vi "Frisbee Joystick.vi"() -> (3 "Value":bool)   [LabVIEW 2012]
uses:
  Users/developer/Desktop/Post TCNJ/Robot Global Data.vi
panel:
  out "s? t:f":dbl
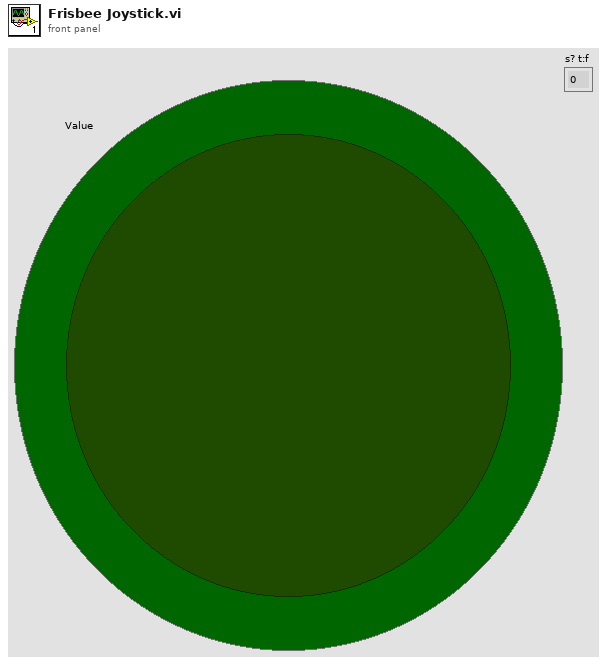
[diagram p1: front panel]
types:
  T1 = cluster{"Driver Station Digital Input (1-8)[0]":bool, "Driver Station Digital Input (1-8)[1]":bool, "Driver Station Digital Input (1-8)[2]":bool, "Driver Station Digital Input (1-8)[3]":bool, "Driver Station Digital Input (1-8)[4]":bool, "Driver Station Digital Input (1-8)[5]":bool, "Driver Station Digital Input (1-8)[6]":bool, "Driver Station Digital Input (1-8)[7]":bool, "Driver Station Digital Input (1-8)[8]":bool}
  T2 = typedef "WPI_DigitalInputDevRef.ctl" = cluster{"DevStatus":errorcluster, "DIO Channel":T3, "Digital Module":T4}
  T3 = typedef "FPGA_DIOChannel.ctl" = enum8{"DIO 1", "DIO 2", "DIO 3", "DIO 4", "DIO 5", "DIO 6", "DIO 7", "DIO 8", "DIO 9", "DIO 10", "DIO 11", "DIO 12", "DIO 13", "DIO 14", "Invalid"}
  T4 = typedef "FPGA_TypedefDigitalModule.ctl" = enum16{"Digital Module 1", "Digital Module 2"}
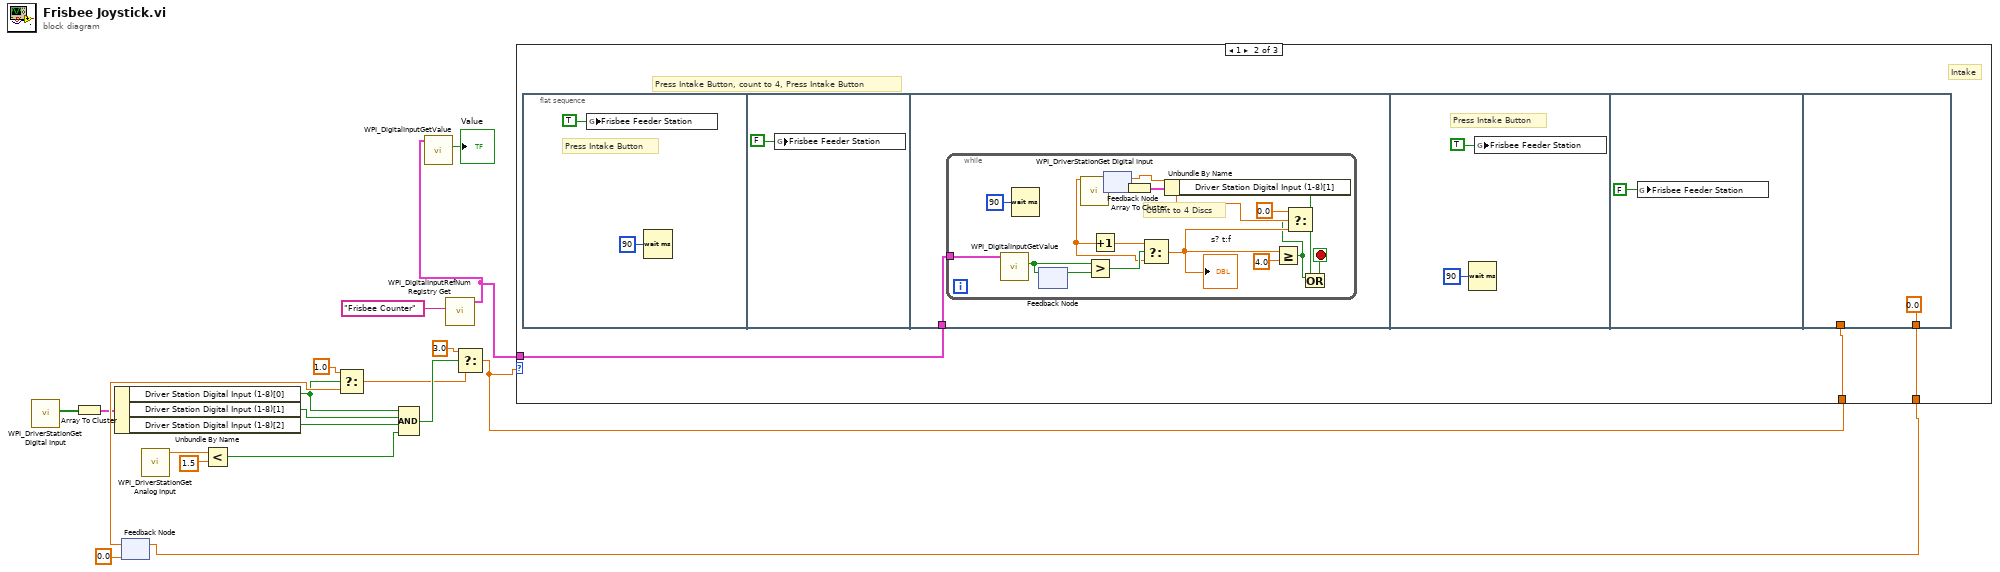
[diagram p0: block diagram]
diagram:
  n1 = call <vilib>:"WPI_DriverStationGet Digital Input.vi"() -> ("Driver Station Digital Input (1-8)"=w4:bool[])  [unwired: 11 in]
  n2 = Array To Cluster(array=w4) -> (cluster=w3:T1)
  n3 = Unbundle By Name(w3) -> ("Driver Station Digital Input (1-8)[0]"=w9:bool, "Driver Station Digital Input (1-8)[1]"=w17:bool, "Driver Station Digital Input (1-8)[2]"=w2:bool)
  n4 = feedback #1(0.0 ("t")) -> (w13:dbl)
  n5 = call <vilib>:"WPI_DriverStationGet Analog Input.vi"() -> ("Analog 1 (V)"=w5:dbl)  [unwired: 8 in, 3 out]
  n6 = Less?(x=w5, y=1.5) -> (x < y?=w7:bool)
  n7 = Select(t=1.0, s=w9, f=w13) -> (s? t:f=w1:dbl)
  n8 = Compound Arithmetic op=AND(w9, w17, w2, w7) -> (w8:bool)
  n9 = call <vilib>:"WPI_DigitalInputRefNum Registry Get.vi"("refnum name"="Frisbee Counter") -> ("DigitalInputDevRef"=w15:T2)  [unwired: 9 in, 1 out]
  n10 = call <vilib>:"WPI_DigitalInputGetValue.vi"("DigitalInputDevRef"=w15) -> ("Value"=→"Value":bool)  [unwired: 8 in, 2 out]
  n11 = Select(t=3.0, s=w8, f=w1) -> (s? t:f=w18:dbl)
  n12 = case shown="1" w18 {
    tunnel: w15 -> [_ w23 _]
    tunnel: w18 -> [w20 w22 w48]
    tunnel: [w20 w21 w48] -> w19
    frame 0, Default {
      # "Waiting For Signal."
      # "Do Nothing"
    }
    frame 1 {
      # "Press Intake Button, count to 4, Press Intake Button"
      # "Intake"
      n13 = flat-sequence {
        tunnel: w23 -> [w27]
        tunnel: w22 -> [_]
        tunnel: [0.0 ("t")] -> w21
        frame #0 {
          # "Press Intake Button"
          n14 = global write "Robot Global Data.vi" "Frisbee Feeder Station"(TRUE) -> ()
          n15 = Wait (ms)(milliseconds to wait=u32 90) -> ()  [unwired: 1 out]
        }
        frame #1 {
          n16 = global write "Robot Global Data.vi" "Frisbee Feeder Station"(FALSE) -> ()
        }
        frame #2 {
          n17 = while {
            tunnel: w27 -> [w39]
            stop <- w28 stop-if-true
            # "Count to 4 Discs"
            n18 = call <vilib>:"WPI_DigitalInputGetValue.vi"("DigitalInputDevRef"=w39) -> ("Value"=w40:bool)  [unwired: 8 in, 2 out]
            n19 = Wait (ms)(milliseconds to wait=u32 90) -> ()  [unwired: 1 out]
            n20 = feedback #2() -> (w41:bool)  [unwired: 1 in]
            n21 = feedback-in #2(w40) -> ()
            n22 = call <vilib>:"WPI_DriverStationGet Digital Input.vi"() -> ("Driver Station Digital Input (1-8)"=w32:bool[])  [unwired: 11 in]
            n23 = Greater?(x=w40, y=w41) -> (0:w43:bool)
            n24 = feedback #3() -> (w36:dbl)  [unwired: 1 in]
            n25 = Increment(x=w36) -> (x+1=w42:dbl)
            n26 = Array To Cluster(array=w32) -> (cluster=w31:T1)
            n27 = Select(t=w42, s=w43, f=w36) -> (s? t:f=w35:dbl)
            "s? t:f" <- w35
            n28 = Unbundle By Name(w31) -> ("Driver Station Digital Input (1-8)[1]"=w29:bool)
            n29 = Greater Or Equal?(x=w35, y=4.0) -> (x >= y?=w30:bool)
            n30 = Select(t=0.0, s=w30, f=w35) -> (s? t:f=w33:dbl)
            n31 = feedback-in #3(w33) -> ()
            n32 = Or(x=w30, y=w29) -> (x .or. y?=w28:bool)
          }
        }
        frame #3 {
          # "Press Intake Button"
          n33 = Wait (ms)(milliseconds to wait=u32 90) -> ()  [unwired: 1 out]
          n34 = global write "Robot Global Data.vi" "Frisbee Feeder Station"(TRUE) -> ()
        }
        frame #4 {
          n35 = global write "Robot Global Data.vi" "Frisbee Feeder Station"(FALSE) -> ()
        }
        frame #5 {
        }
      }
    }
    frame 3 {
      # "Harlem Shake"
    }
  }
  n36 = feedback-in #1(w19) -> ()
